vi "Connect Timeout.vi"(8 "error in (no error)":errorcluster, 9 "connect_timeout_ms":u64, 11 "ClientBuilder in":refnum<class "ClientBuilder.lvclass">) -> (0 "error out":errorcluster, 2 "success":bool, 3 "ClientBuilder out":refnum<class "ClientBuilder.lvclass">)   [LabVIEW 2020, in "reqwest.lvlib" / "ClientBuilder.lvclass"]
uses:
  ClientBuilder.lvclass
  ClientBuilder.lvclass/ClientBuilder.ctl
  lv_reqwest_64.dll
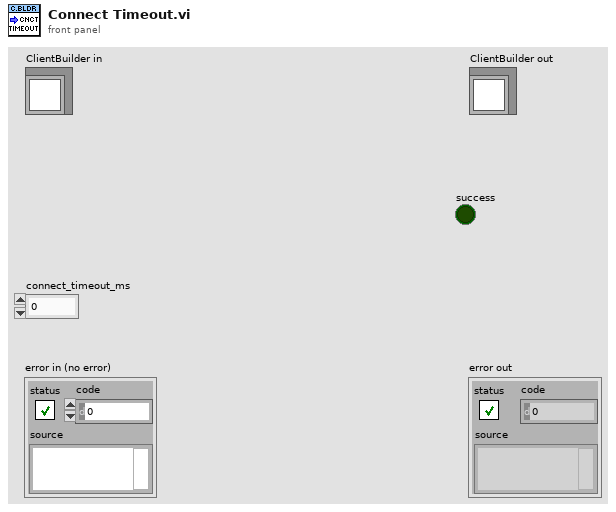
[diagram p1: front panel]
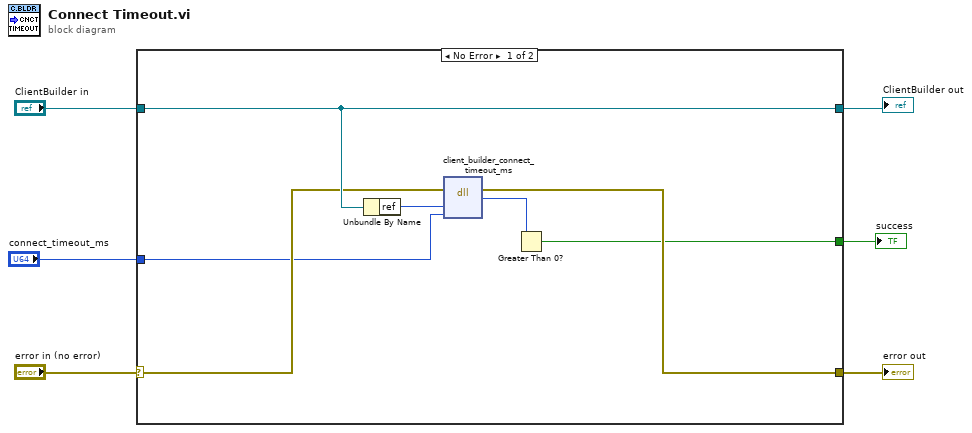
[diagram p0: block diagram]
diagram:
  n1 = case shown="No Error" "error in (no error)" {
    selector: "error in (no error)" -> [w10 w14]
    tunnel: "ClientBuilder in" -> [w11 w15]
    tunnel: [w13 w14] -> w3
    tunnel: [w11 w15] -> w4
    tunnel: "connect_timeout_ms" -> [w9 _]
    tunnel: [w7 _] -> w1
    frame No Error {
      n2 = Unbundle By Name(w11) -> ("ref"=w12:u64)
      n3 = dll-call lib="C:/Projects/reqwest-rs-labview/lv_src/lv_reqwest_*.*" fn="client_builder_connect_timeout_ms"(error in=w10, "client_builder_ref"=w12, "timeout_ms"=w9) -> (error out=w13:errorcluster, "success"=w8:u8)  [unwired: 4 in, 1 out]
      n4 = Greater Than 0?(x=w8) -> (x > 0?=w7:bool)
    }
    frame Error {
    }
  }
  "error out" <- w3
  "ClientBuilder out" <- w4
  "success" <- w1
